vi "RX_basic.vi"() -> ()   [LabVIEW 2013]
uses:
  <vilib>/sound2/lvsound2.llb/Sound Data Format.ctl
  <instrlib>/niUSRP/niUSRP Fetch Rx Data (CDB WDT).vi
  <vilib>/Analysis/2dsp.llb/Rational Resample (single channel, DBL).vi
  <vilib>/sound2/lvsound2.llb/Sound Output Write (DBL Single).vi
  <vilib>/express/express analysis/Spectral/Block/exnSpectralBlock spectral measurements RMS poly.vi
  <vilib>/express/express analysis/Spectral/Block/exnSpectralBlock spectral measurements RMS WFM.vi
  <vilib>/express/express analysis/Spectral/XNode/ExpressSpectralMeasurementsBlockNode.xnode
  <vilib>/Analysis/NI_AALPro.lvlib
panel:
  out "XY Graph":cluster{dbl[], dbl[]}(graph)
  out "error out 2":errorcluster
  in  "sound format":T1={"sample rate (S/s)"=44100.0, "number of channels"=1, "bits per sample"=16}
  in  "number of samples":i64=44100
  out "coerced gain":dbl format="%#_6f"
  out "coerced carrier frequency":dbl=2400000000.0 format="%#_6p"
  out "coerced IQ rate":dbl=200000.0 format="%#_6p"
  in  "active antenna":string="RX2"
  in  "gain":dbl format="%#_6f"
  in  "carrier frequency":dbl=2400000000.0 format="%#_6p"
  in  "IQ rate":dbl=200000.0 format="%#_6p"
  out "error out":errorcluster
  in  "device names":refnum<k15>="192.168.10.4"
  in  "stop":bool
  out "Waveform Graph":cluster{"f0":dbl, "df":dbl, "magnitude":dbl[]}(graph)
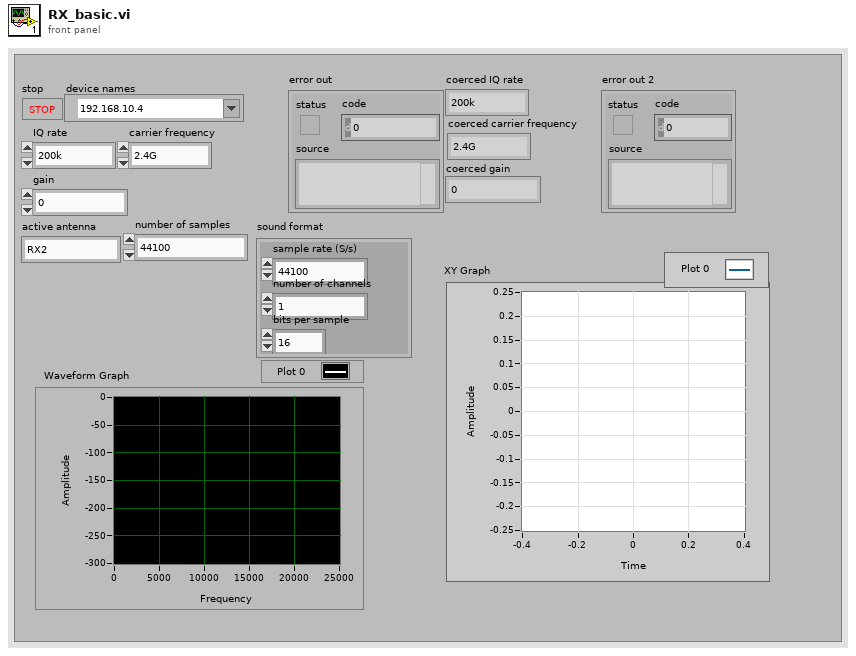
[diagram p1: front panel]
types:
  T1 = typedef "Sound Data Format.ctl" = cluster{"sample rate (S/s)":dbl, "number of channels":i32, "bits per sample":i32}
  T2 = typedef "Sound Output Task ID.ctl" = u32
  T3 = cluster{"averaging mode":u16, "weighting mode":u16, "number of averages":u32}
  T4 = cluster{"dB On (F)":bool, "unwrap phase (F)":bool, "convert to degree (F)":bool}
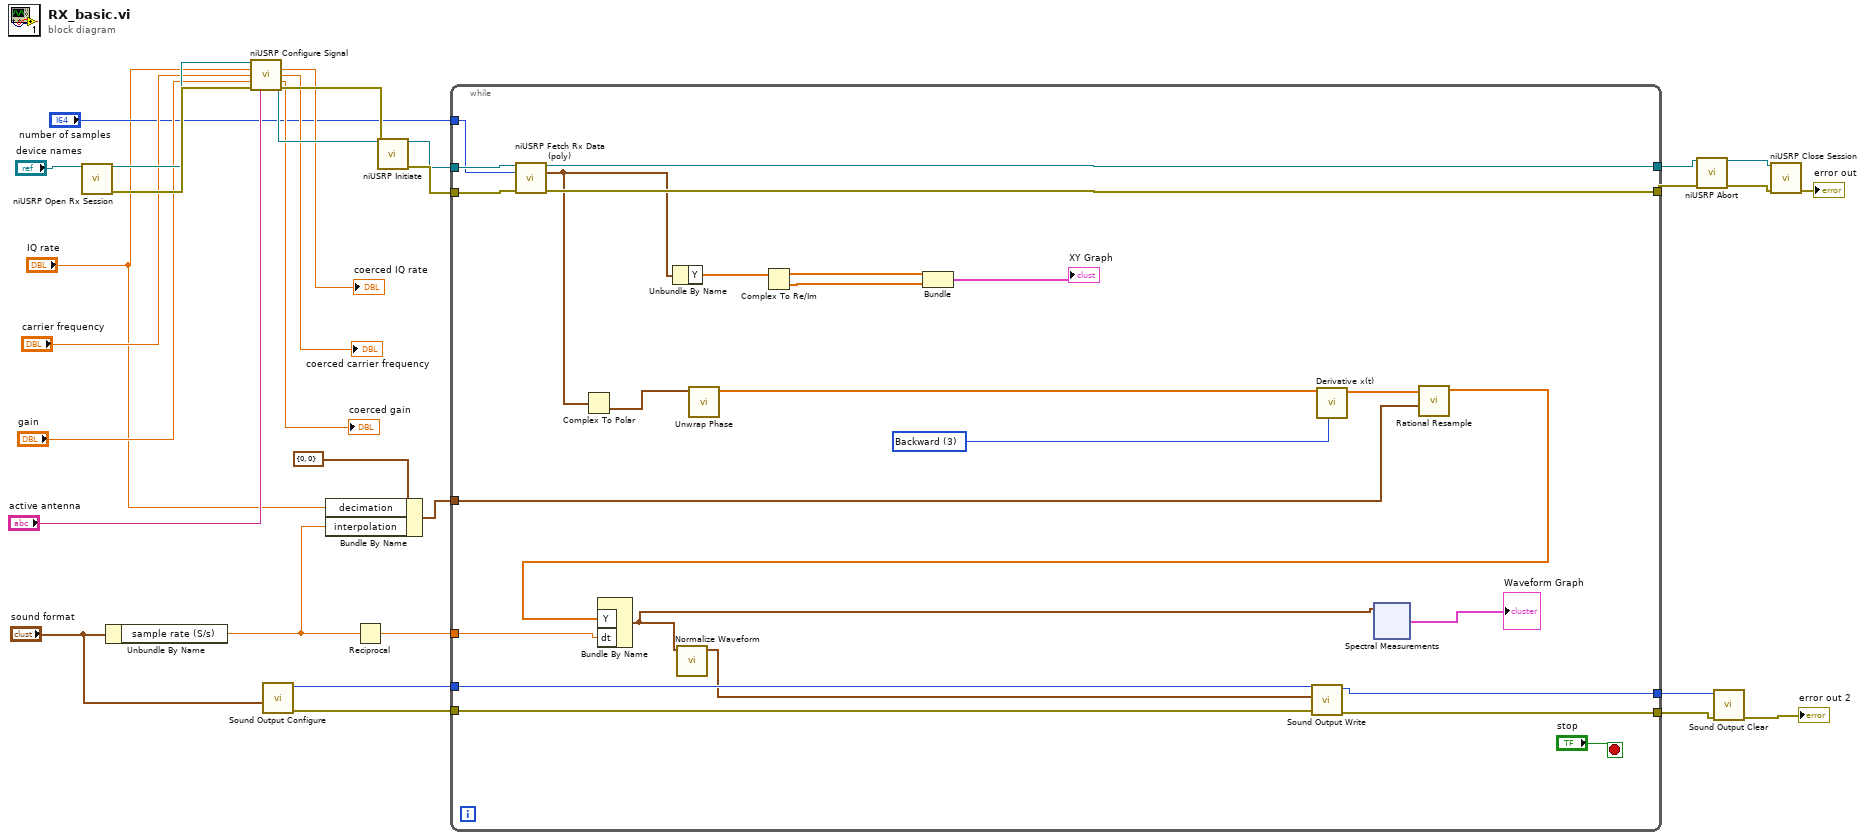
[diagram p0: block diagram]
diagram:
  n1 = call <instrlib>:"niUSRP Open Rx Session.vi"("device names"="device names") -> ("session handle out"=w19:refnum<k15>, "error out"=w29:errorcluster)  [unwired: 13 in]
  n2 = Unbundle By Name("sound format") -> ("sample rate (S/s)"=w9:dbl)
  n3 = call <instrlib>:"niUSRP Configure Signal.vi"("session handle"=w19, "IQ rate"="IQ rate", "carrier frequency"="carrier frequency", "gain"="gain", "error in (no error)"=w29, "active antenna"="active antenna") -> ("session handle out"=w20:refnum<k15>, "coerced IQ rate"=→"coerced IQ rate":dbl, "coerced carrier frequency"=→"coerced carrier frequency":dbl, "coerced gain"=→"coerced gain":dbl, "error out"=w28:errorcluster)  [unwired: 5 in]
  n4 = call <vilib>:"Sound Output Configure.vi"("sound format"="sound format") -> ("error out"=w8:errorcluster, "task ID"=w3:T2)  [unwired: 9 in]
  n5 = Bundle By Name(cluster=cluster{"decimation":i32, "interpolation":i32} {"decimation"=0, "interpolation"=0}, "decimation"="IQ rate", "interpolation"=w9) -> (w4:cluster{"decimation":i32, "interpolation":i32})
  n6 = Reciprocal(x=w9) -> (1/x=w5:dbl)
  n7 = call <instrlib>:"niUSRP Initiate.vi"("session handle"=w20, "error in (no error)"=w28) -> ("session handle out"=w23:refnum<k15>, "error out"=w27:errorcluster)  [unwired: 12 in]
  n8 = while {
    tunnel: w27 -> [w54]
    tunnel: [w53] -> w26
    tunnel: w23 -> [w52]
    tunnel: [w51] -> w22
    tunnel: "number of samples" -> [w50]
    tunnel: w8 -> [w47]
    tunnel: [w46] -> w7
    tunnel: w5 -> [w45]
    tunnel: w4 -> [w44]
    tunnel: w3 -> [w42]
    tunnel: [w41] -> w2
    stop <- "stop" stop-if-true
    w31 = u16 3 items=["2nd Order Central", "4th Order Central", "Forward", "Backward"] ("method")
    n9 = call-poly <instrlib>:"niUSRP Fetch Rx Data (poly).vi"("session handle"=w52, "number of samples"=w50, "error in (no error)"=w54) -> ("session handle out"=w51:refnum<k15>, "data"=w37:waveform(cdb), "error out"=w53:errorcluster)  [unwired: 9 in, 1 out]
    n10 = Complex To Polar(r * e^(i*theta)=w37) -> (theta=w36:waveform(dbl))  [unwired: 1 out]
    n11 = Unbundle By Name(w37) -> ("Y"=w35:cdb[])
    n12 = call <vilib>:"Unwrap Phase.vi"("Phase"=w36) -> ("Unwrapped Phase"=w49:dbl[])  [unwired: 9 in, 1 out]
    n13 = Complex To Re/Im(x + iy=w35) -> (x=w34:dbl[], y=w33:dbl[])
    n14 = Bundle(w34, w33) -> (→"XY Graph":cluster{dbl[], dbl[]})  [unwired: 1 in]
    n15 = call <vilib>:"Derivative x(t).vi"("method"=w31, "X"=w49) -> ("dX/dt"=w48:dbl[])  [unwired: 8 in, 1 out]
    n16 = call-poly <vilib>:"Rational Resample.vi"("resample factor"=w44, "X"=w48) -> ("Y"=w43:dbl[])  [unwired: 7 in, 2 out]
    n17 = Bundle By Name("Y"=w43, "dt"=w45) -> (w39:waveform(dbl))  [unwired: 1 in]
    n18 = call <vilib>:"Normalize Waveform.vi"("waveform in"=w39) -> ("normalized waveform"=w40:waveform(dbl))  [unwired: 7 in, 3 out]
    n19 = call-poly <vilib>:"Sound Output Write.vi"("error in (no error)"=w47, "data"=w40, "task ID"=w42) -> ("error out"=w46:errorcluster, "task ID out"=w41:T2)  [unwired: 7 in]
    n20 = xnode ("Spectral Measurements")("Signals"=w39) -> ("FFT - (RMS)"=→"Waveform Graph":cluster{"f0":dbl, "df":dbl, "magnitude":dbl[]})  [unwired: 1 in, 2 out]
  }
  n21 = call <instrlib>:"niUSRP Abort.vi"("session handle"=w22, "error in (no error)"=w26) -> ("session handle out"=w21:refnum<k15>, "error out"=w25:errorcluster)  [unwired: 12 in]
  n22 = call <vilib>:"Sound Output Clear.vi"("error in (no error)"=w7, "task ID"=w2) -> ("error out"=→"error out 2":errorcluster)  [unwired: 9 in]
  n23 = call <instrlib>:"niUSRP Close Session.vi"("session handle"=w21, "error in (no error)"=w25) -> ("error out"=→"error out":errorcluster)  [unwired: 13 in]
